vi "Connect to WiFi network.vi"() -> ()   [LabVIEW 2016]
uses:
  VISA resource XBee.vi
panel:
  out "x/y":dbl
  out "WiFi Networks":string[][](table)
  out "Latest AT command response":string
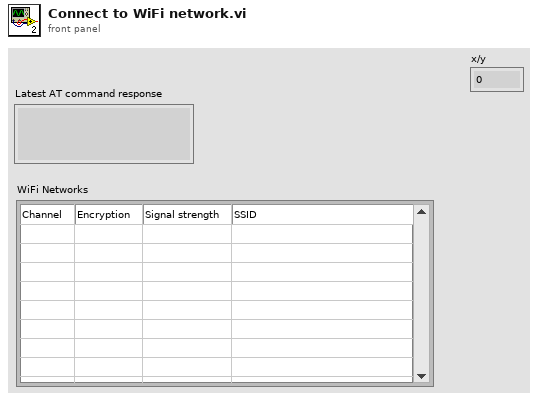
[diagram p1: front panel]
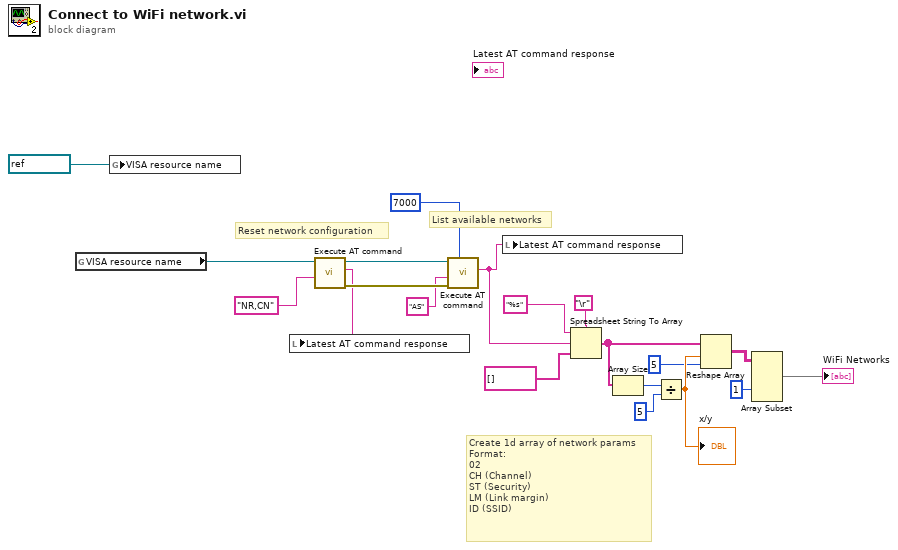
[diagram p0: block diagram]
diagram:
  # "Create 1d array of network params\nFormat:\n02\nCH (Channel)\nST (Security)\nLM (Link margin)\nID (SSID)"
  # "List available networks"
  # "Reset network configuration"
  n1 = global read "VISA resource XBee.vi" "VISA resource name"() -> (w20:refnum<visa-resource-name>)
  n2 = global write "VISA resource XBee.vi" "VISA resource name"(refnum<visa-resource-name> "COM4" ("VISA resource name")) -> ()
  n3 = call "Execute AT command.vi"("AT Command"="NR,CN", "VISA resource in"=w20) -> ("error out"=w17:errorcluster, "Response message"=w14:string, "VISA resource out"=w18:refnum<visa-resource-name>)  [unwired: 6 in]
  n4 = local write "Latest AT command response"(w14) -> ()
  n5 = call "Execute AT command.vi"("milliseconds to wait"=u32 7000, "error in (no error)"=w17, "AT Command"="AS", "VISA resource in"=w18) -> ("Response message"=w7:string)  [unwired: 4 in, 2 out]
  n6 = local write "Latest AT command response"(w7) -> ()
  n7 = Spreadsheet String To Array(delimiter (Tab)="\r", format string="%s" ("spreadsheet string"), spreadsheet string=w7, array type (2D Dbl)=string[] []) -> (array=w2:string[])
  n8 = Array Size(array=w2) -> (size(s)=w11:i32)
  n9 = Divide(x=w11, y=5) -> (x/y=w9:dbl)
  "x/y" <- w9
  n10 = Reshape Array(w2, w9, 5 ("dimension size")) -> (w4:string[][])
  n11 = Array Subset(array=w4, index (col)=1 ("index")) -> (→"WiFi Networks":string[][])  [unwired: 3 in]
